vi "Control Arduino.vi"() -> ()   [LabVIEW 2021]
uses:
  <vilib>/Instr/_visa.llb/VISA Configure Serial Port (Instr).vi
panel:
  in  "VISA resource name":refnum<visa-resource-name>
  in  "LED":bool
  in  "Stop Button":bool
  # "1. Select the serial port (VISA resource name)\n2. Use the LED button to control the Arduino's board LED\n3. Use the Stop button to stop the program"
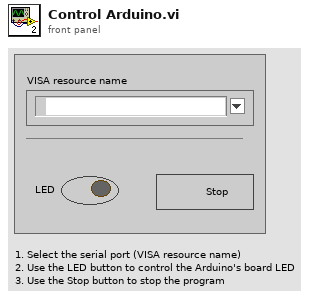
[diagram p1: front panel]
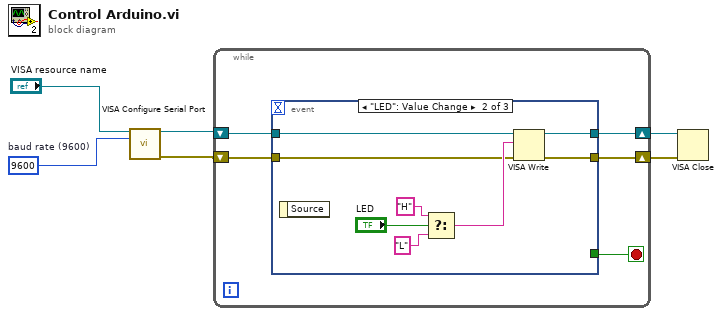
[diagram p0: block diagram]
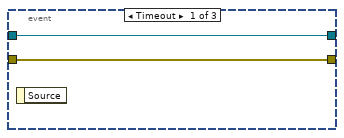
[diagram p2: hidden frame]
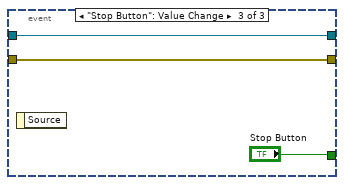
[diagram p3: hidden frame]
diagram:
  w6 = u32 9600  # baud rate (9600)
  n1 = call-poly "VISA Configure Serial Port"("VISA resource name"="VISA resource name", "baud rate (9600)"=w6) -> ("VISA resource name out"=w4:refnum<visa-resource-name>, "error out"=w2:errorcluster)  [unwired: 12 in]
  n2 = while {
    shift-right: [w8] -> w3
    shift-left: w4 -> [w9]
    shift-right: [w7] -> w5
    shift-left: w2 -> [w10]
    stop <- w11 stop-if-true
    n3 = event shown="[1] \"LED\": Value Change" {
      selector: _ -> [_ _ _]
      dyn-events: _ -> [_ _ _]
      timeout: _ -> [_ _ _]
      tunnel: [_ _ "Stop Button"] -> w11
      tunnel: w10 -> [w12 w17 w22]
      tunnel: w9 -> [w13 w16 w23]
      tunnel: [w13 w15 w23] -> w8
      tunnel: [w12 w14 w22] -> w7
      event Timeout {
        n4 = event-data() -> ()  [unwired: 1 in, 1 out]
      }
      event "LED": Value Change {
        n5 = event-data() -> ()  [unwired: 1 in, 1 out]
        n6 = Select(t="H", s="LED", f="L") -> (s? t:f=w20:string)
        n7 = VISA Write(VISA resource name=w16, write buffer=w20, error in (no error)=w17) -> (VISA resource name out=w15:refnum<visa-resource-name>, error out=w14:errorcluster)  [unwired: 1 out]
      }
      event "Stop Button": Value Change {
        n8 = event-data() -> ()  [unwired: 1 in, 1 out]
      }
    }
  }
  n9 = VISA Close(VISA resource name=w3, error in (no error)=w5) -> ()  [unwired: 1 out]
